vi "AFM_TF_control.vi"() -> ()   [LabVIEW 2017]
uses:
  controls/ControlParams_TF.ctl
  <vilib>/rvi/Emulation/niFpgaGetClockAttributes.vi
  <vilib>/rvi/Emulation/niFpgaSctlEmulationGetInTimedLoop.vi
  <vilib>/rvi/Emulation/niFpgaEmulationReportErrorSimple.vi
  <vilib>/rvi/eio/common/nirviEmuTemplateMethod_errors.vi
  <vilib>/rvi/Emulation/niFpgaCriticalErrorInLSC.vi
  <vilib>/rvi/Emulation/niFpgaProcessEmulError.vi
  <vilib>/rvi/interface/RandomDataEmulation/niFpgaRandomDataHandleErrors.vi
  <vilib>/eio/EIONode/EIONode.xnode
  <vilib>/rvi/DataTransferAndStorage/Container/XNode/niFpgaContainer.xnode
  <vilib>/rvi/interface/RandomDataEmulation/nirviRandomDataFpgaReadWriteTemplate.vi
  <vilib>/rvi/FXPMathLib/FxpSub/XNode/nifxpmath_Sub.xnode
  <vilib>/rvi/FXPMathLib/sim/FxpSim.dll
panel:
  out "TF Order":u8
  in  "ControlParams":T1={"Umax "=0.0, "ymax"=0.0, "TsTicks"=0, "num"=[0.0, 0.0, 0.0, 0.0, 0.0, 0.0, 0.0, 0.0, 0.0], "den"=[0.0, 0.0, 0.0, 0.0, 0.0, 0.0, 0.0, 0.0, 0.0], "TF Order"=0, "num_ff"=[0.0, 0.0, 0.0, 0.0, 0.0, 0.0, 0.0, 0.0, 0.0], "den_ff"=[0.0, 0.0, 0.0, 0.0, 0.0, 0.0, 0.0, 0.0, 0.0], "TF_ff_order "=0, "ff_on"=FALSE}
  out "yref_k":sgl
  out "yuxk TO":bool
  out "YK TO":bool
  out "Unstable Traj":bool
  out "Loop Done":bool
  in  "Settle Ticks":i16=1000
  in  "Abort":bool=TRUE
  in  "iters":i16=1
  in  "ymax":sgl=4.0 format="%#_13g"
  out "TsTicks":i16
  out "Loop Ticks (benchmark)":i16
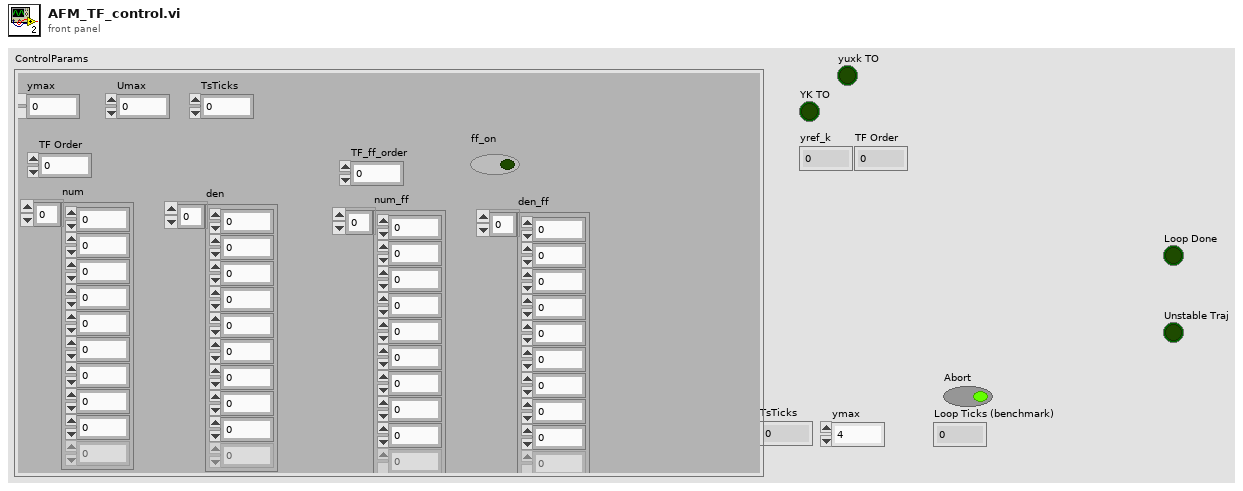
[diagram p1: front panel]
types:
  T1 = typedef "ControlParams_TF.ctl" = cluster{"Umax ":sgl, "ymax":sgl, "TsTicks":u32, "num":sgl[], "den":sgl[], "TF Order":u8, "num_ff":sgl[], "den_ff":sgl[], "TF_ff_order ":u8, "ff_on":bool}
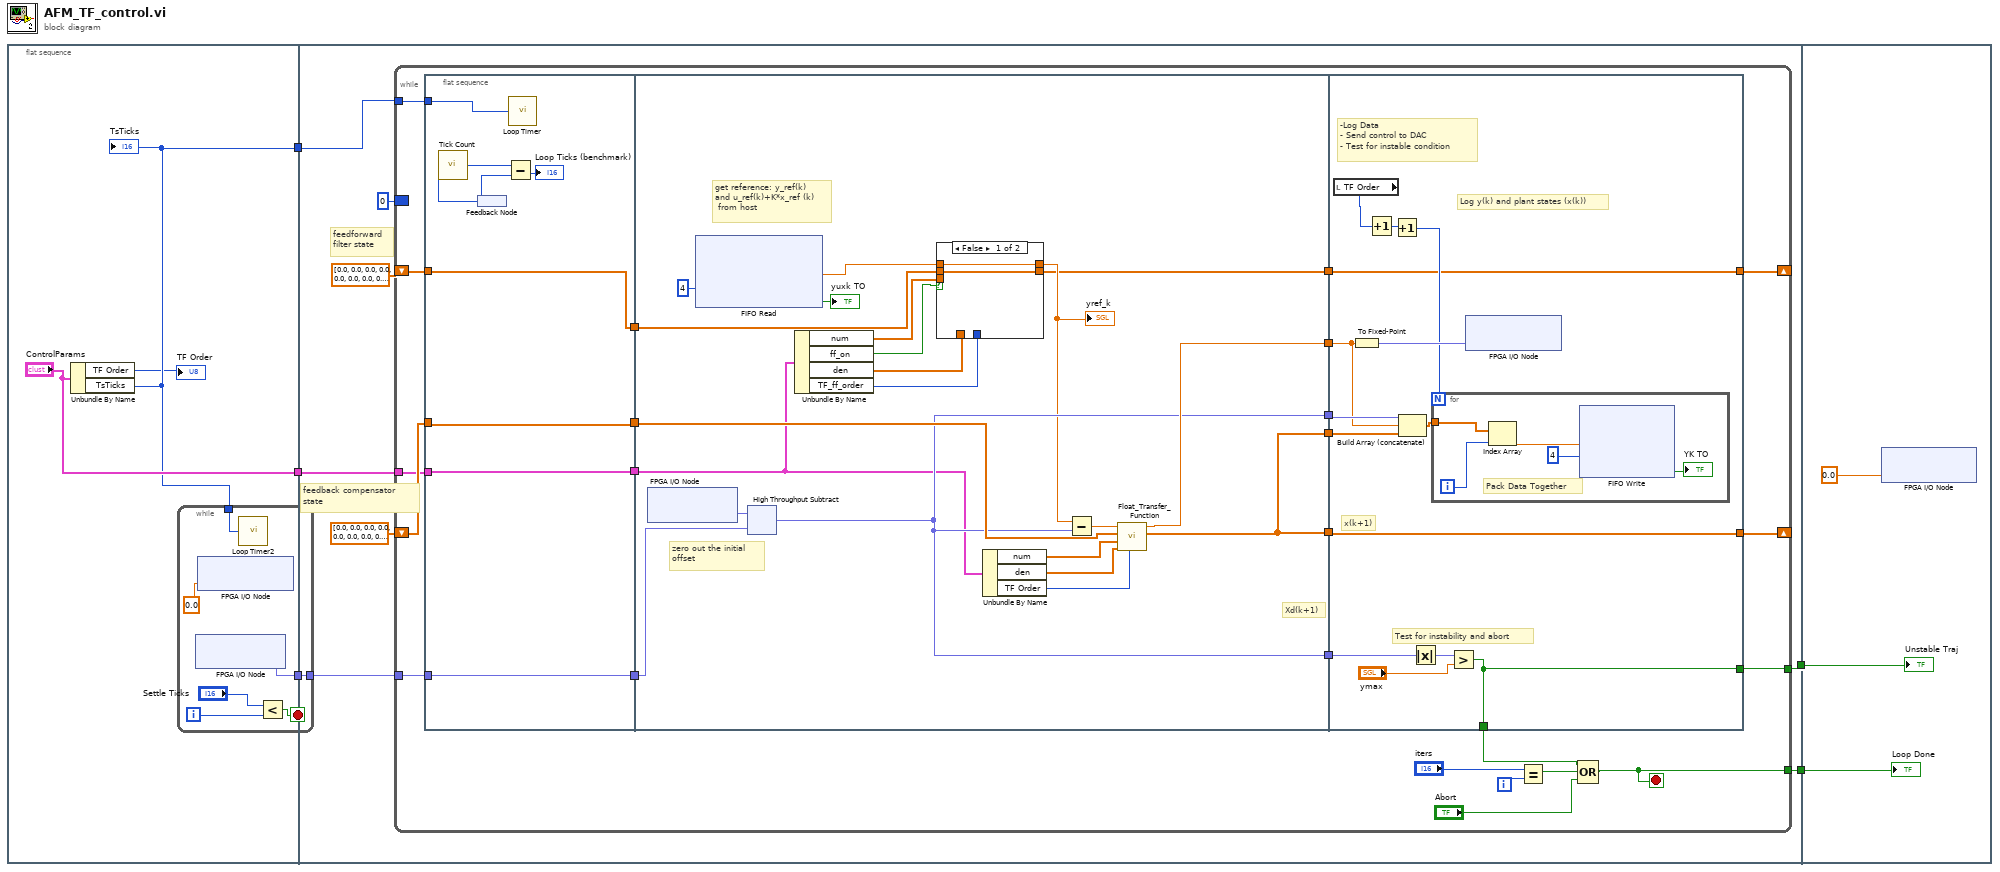
[diagram p0: block diagram]
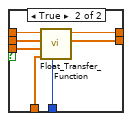
[diagram p2: hidden frame]
diagram:
  n1 = flat-sequence {
    tunnel: [w7] -> w5
    tunnel: [w9] -> w4
    tunnel: ["ControlParams"] -> w2
    tunnel: w5 -> [w22]
    tunnel: w4 -> [w21]
    tunnel: [w19] -> w3
    tunnel: w2 -> [w18]
    tunnel: [w17] -> w1
    tunnel: w3 -> [w106]
    tunnel: w1 -> [w105]
    frame #0 {
      # "Load Matrix Data"
      n2 = Unbundle By Name("ControlParams") -> ("TF Order"=→"TF Order":u8, "TsTicks"=w7:u32)
      "TsTicks" <- w7
      n3 = while {
        tunnel: [w15] -> w9
        tunnel: w7 -> [w14]
        i -> [w10]
        stop <- w12 stop-if-true
        n4 = xnode "FPGA I/O Node"() -> ("Mod2/AI0"=w15:fxp<+/-,24,5>)  [unwired: 1 in, 1 out]
        n5 = xnode "FPGA I/O Node"("Mod1/AO0"=sgl 0.0) -> ()  [unwired: 1 in, 1 out]
        n6 = call "Loop Timer2"("Count(Ticks)"=w14) -> ()  [unwired: 1 out]
        n7 = Less?(x="Settle Ticks", y=w10) -> (x < y?=w12:bool)
      }
    }
    frame #1 {
      # "feedback compensator \nstate"
      # "feedforward\nfilter state"
      n8 = while {
        border: i16 0 -> [_]
        tunnel: w22 -> [w45]
        tunnel: w21 -> [w43]
        shift-right: [w33] -> _
        shift-left: sgl[] [0.0, 0.0, 0.0, 0.0, 0.0, 0.0, 0.0, 0.0, 0.0] ("x^(k+1) = Ax + Bu + Lye") -> [w41]
        tunnel: [w28] -> w19
        tunnel: w18 -> [w38]
        tunnel: [w37] -> w17
        shift-right: [w26] -> _
        shift-left: sgl[] [0.0, 0.0, 0.0, 0.0, 0.0, 0.0, 0.0, 0.0, 0.0] ("x^(k+1) = Ax + Bu + Lye") -> [w25]
        i -> [w46]
        stop <- w28 stop-if-true
        n9 = flat-sequence {
          tunnel: w45 -> [w52]
          tunnel: w43 -> [w51]
          tunnel: [w51] -> w42
          tunnel: w41 -> [w49]
          tunnel: [w49] -> w40
          tunnel: [w50] -> w39
          tunnel: w38 -> [w50]
          tunnel: w25 -> [w48]
          tunnel: [w48] -> w24
          tunnel: [w68] -> w44
          tunnel: w42 -> [w76]
          tunnel: w40 -> [w73]
          tunnel: w39 -> [w62]
          tunnel: [w68] -> w36
          tunnel: [w72] -> w35
          tunnel: [w67] -> w34
          tunnel: [w67] -> w32
          tunnel: [w63] -> w27
          tunnel: w24 -> [w59]
          tunnel: [w93] -> w30
          tunnel: w44 -> [w96]
          tunnel: [w93] -> w37
          tunnel: w36 -> [w92]
          tunnel: w35 -> [w88]
          tunnel: w34 -> [w89]
          tunnel: [w87] -> w33
          tunnel: w32 -> [w87]
          tunnel: [w86] -> w26
          tunnel: w27 -> [w86]
          frame #0 {
            n10 = call "Tick Count"() -> ("Tick Count(Ticks)"=w53:u32)
            n11 = feedback #1() -> (w54:u32)
            n12 = feedback-in #1(w53) -> ()
            n13 = Subtract(x=w53, y=w54) -> (x-y=→"Loop Ticks (benchmark)":u32)
            n14 = call "Loop Timer"("Count(Ticks)"=w52) -> ()  [unwired: 1 out]
          }
          frame #1 {
            # "get reference: y_ref(k)\nand u_ref(k)+K*x_ref (k)\n from host"
            # "Xd(k+1)"
            # "zero out the initial \noffset"
            n15 = xnode "FPGA I/O Node"() -> ("Mod2/AI0"=w75:fxp<+/-,24,5>)  [unwired: 1 in, 1 out]
            n16 = xnode ("FIFO Read")("Timeout"=i16 4) -> ("Element"=w60:sgl, "Timed Out?"=→"yuxk TO":bool)  [unwired: 1 in, 1 out]
            n17 = xnode "High Throughput Subtract"("x"=w75, "y"=w76) -> ("x-y"=w68:fxp<+/-,40,6>)
            n18 = Unbundle By Name(w62) -> ("num"=w58:sgl[], "ff_on"=w56:bool, "den"=w57:sgl[], "TF_ff_order"=w61:u8)
            n19 = case shown="False" w56 {
              tunnel: [w78 w85] -> w64
              tunnel: [w77 w84] -> w63
              tunnel: w58 -> [_ w83]
              tunnel: w57 -> [_ w82]
              tunnel: w61 -> [_ w81]
              tunnel: w60 -> [w78 w80]
              tunnel: w59 -> [w77 w79]
              frame False {
              }
              frame True {
                n20 = call "Float_Transfer_Function.vi"("TF Order"=w81, "Den"=w82, "Num"=w83, "State In"=w79, "Input"=w80) -> ("State Out"=w84:sgl[], "Output"=w85:sgl)  [unwired: 4 in]
              }
            }
            "yref_k" <- w64
            n21 = Unbundle By Name(w62) -> ("num"=w69:sgl[], "den"=w70:sgl[], "TF Order"=w71:u8)
            n22 = Subtract(x=w64, y=w68) -> (x-y=w74:sgl)
            n23 = call "Float_Transfer_Function.vi"("TF Order"=w71, "Den"=w70, "Num"=w69, "State In"=w73, "Input"=w74) -> ("State Out"=w67:sgl[], "Output"=w72:sgl)  [unwired: 4 in]
          }
          frame #2 {
            # "x(k+1)"
            # "Log y(k) and plant states (x(k))"
            # "-Log Data\n- Send control to DAC\n- Test for instable condition"
            # "Test for instability and abort"
            n24 = local read "TF Order"() -> (w95:u8)
            n25 = To Fixed-Point(number=w88) -> (fixed-point=w94:fxp<+/-,32,6>)  [unwired: 1 in]
            n26 = Increment(x=w95) -> (x+1=w91:u8)
            n27 = Increment(x=w91) -> (x+1=w90:u8)
            n28 = Build Array (concatenate)(w96, w88, w89) -> (w97:sgl[])
            n29 = Absolute Value(x=w92) -> (abs(x)=w99:fxp<+,40,6>)
            n30 = for {
              N: w90 -> [_]
              tunnel: w97 -> [w102]
              i -> [w103]
              # "Pack Data Together"
              n31 = Index Array(array=w102, index=w103) -> (element=w101:sgl)
              n32 = xnode ("FIFO Write")("Element"=w101, "Timeout"=i16 4) -> ("Timed Out?"=→"YK TO":bool)  [unwired: 1 in, 1 out]
            }
            n33 = Greater?(x=w99, y="ymax") -> (0:w93:bool)
            n34 = xnode "FPGA I/O Node"("Mod1/AO0"=w94) -> ()  [unwired: 1 in, 1 out]
          }
        }
        n35 = Equal?(x="iters", y=w46) -> (x = y?=w31:bool)
        n36 = Compound Arithmetic op=OR(w30, w31, "Abort") -> (w28:bool)
      }
    }
    frame #2 {
      n37 = xnode "FPGA I/O Node"("Mod1/AO0"=sgl 0.0) -> ()  [unwired: 1 in, 1 out]
      "Loop Done" <- w106
      "Unstable Traj" <- w105
    }
  }
